vi "Write Multiplicator.vi"(8 "error in (no error)":errorcluster, 10 "Multiplicator":dbl=1.0, 11 "TG Base Graph in":refnum<class "TG Base Graph.lvclass">) -> (0 "error out":errorcluster, 3 "TG Base Graph out":refnum<class "TG Base Graph.lvclass">)   [LabVIEW 2023]
uses:
  TG Base Graph.lvclass
  TG Base Graph.lvclass/TG Base Graph.ctl
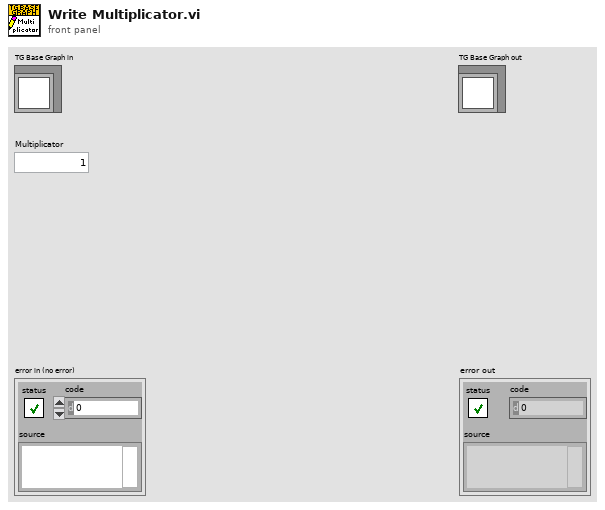
[diagram p1: front panel]
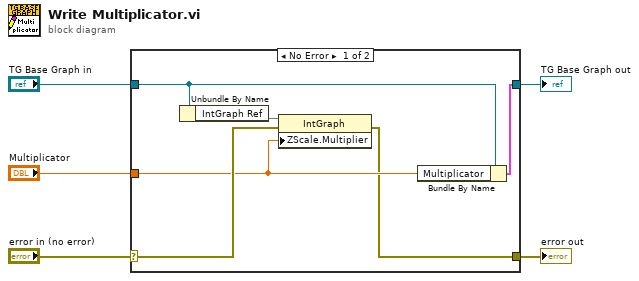
[diagram p0: block diagram]
diagram:
  n1 = case shown="No Error" "error in (no error)" {
    selector: "error in (no error)" -> [w8 w12]
    tunnel: [w6 w12] -> w4
    tunnel: [w11 w13] -> w2
    tunnel: "TG Base Graph in" -> [w10 w13]
    tunnel: "Multiplicator" -> [w7 _]
    frame No Error {
      n2 = Unbundle By Name(w10) -> ("IntGraph Ref"=w9)
      n3 = property class="IntGraph"(reference=w9, error in=w8, "ZScale.Multiplier"=w7) -> (error out=w6:errorcluster)  [unwired: 1 out]
      n4 = Bundle By Name(cluster=w10, "Multiplicator"=w7) -> (w11:cluster{})
    }
    frame Error {
    }
  }
  "error out" <- w4
  "TG Base Graph out" <- w2
